vi "testDataPass_v2,0_vi0.vi"() -> ()   [LabVIEW 2014]
uses:
  testDataPass_v2,0_global1.vi
panel:
  in  "stop":bool
  out "error out 2":errorcluster
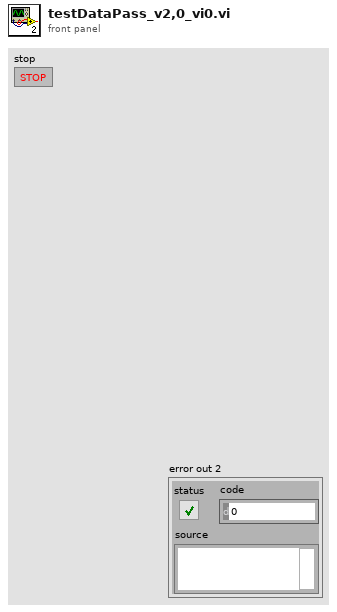
[diagram p1: front panel]
types:
  T1 = enum32{"Invalid", "Standard", "Closed", "Hidden", "Minimized", "Maximized"}
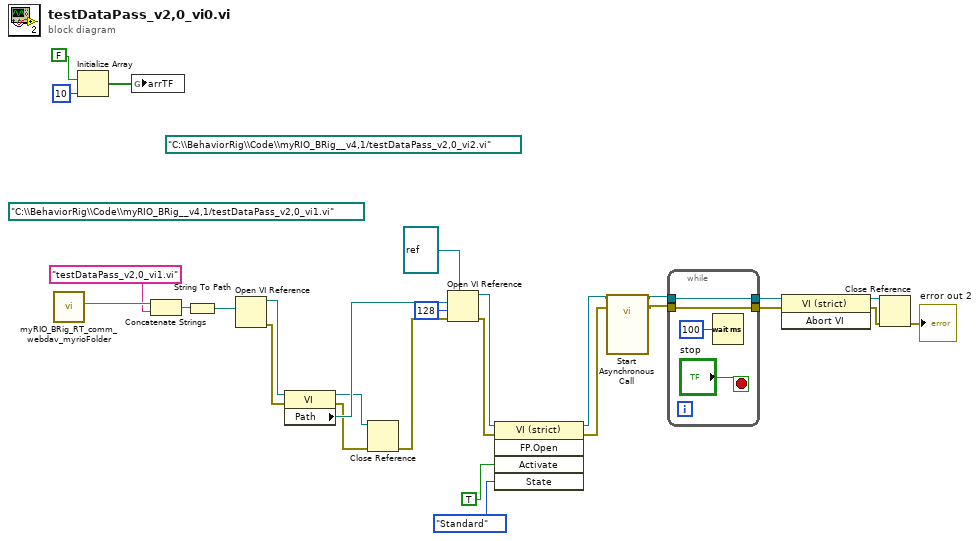
[diagram p0: block diagram]
diagram:
  (unwired) path "C:\\BehaviorRig\\Code\\myRIO_BRig__v4,1/testDataPass_v2,0_vi1.vi" ("vi path")
  (unwired) path "C:\\BehaviorRig\\Code\\myRIO_BRig__v4,1/testDataPass_v2,0_vi2.vi" ("vi path")
  n1 = call "myRIO_BRig_RT_comm_webdav_myrioFolder.vi"() -> ("output_myrioFolder"=w28:string)  [unwired: 11 in]
  n2 = Initialize Array(FALSE, 10 ("dimension size")) -> (w26:bool[])
  n3 = global write "testDataPass_v2,0_global1.vi" "arrTF"(w26) -> ()
  n4 = Concatenate Strings(w28, "testDataPass_v2,0_vi1.vi" ("string")) -> (w21:string)
  n5 = String To Path(string=w21) -> (path=w13:path)
  n6 = Open VI Reference(vi path=w13) -> (vi reference=w12:refnum<vi>, error out=w11:errorcluster)  [unwired: 5 in]
  n7 = property class="VI"(reference=w12, error in=w11) -> (reference out=w9:refnum<vi>, error out=w8:errorcluster, "Path"=w10:path)
  n8 = Close Reference(reference=w9, error in (no error)=w8) -> (error out=w7:errorcluster)
  n9 = Open VI Reference(type specifier VI Refnum (for type only)=refnum<vi> refnum, vi path=w10, options=128, error in (no error)=w7) -> (vi reference=w6:refnum<vi>, error out=w5:errorcluster)  [unwired: 2 in]
  n10 = invoke class="VI (strict)" method="FP.Open"(reference=w6, error in=w5, "Activate"=TRUE ("Activate?"), "State"=T1."Standard") -> (reference out=w4:refnum<vi>, error out=w3:errorcluster)  [unwired: 1 in, 3 out]
  n11 = call-by-ref "Start Asynchronous Call"(reference=w4, error in=w3) -> (reference out=w1:refnum<vi>, error out=w2:errorcluster)  [unwired: 12 in]
  n12 = while {
    tunnel: w1 -> [w30]
    tunnel: w2 -> [w29]
    tunnel: [w30] -> w17
    tunnel: [w29] -> w16
    stop <- "stop" stop-if-true
    n13 = Wait (ms)(milliseconds to wait=u32 100) -> ()  [unwired: 1 out]
  }
  n14 = invoke class="VI (strict)" method="Abort VI"(reference=w17, error in=w16) -> (reference out=w15:refnum<vi>, error out=w14:errorcluster)  [unwired: 1 in, 1 out]
  n15 = Close Reference(reference=w15, error in (no error)=w14) -> (error out=→"error out 2":errorcluster)
